vi "Settings Dialog.vi"(11 "settings in":T1={"sample rate"=100.0, "input range"=10.0, "logfile path"=path "", "Simulated Signal"={"signal type"=enum."Sine Wave", "frequency"=1000.0, "amplitude"=5.0}} {"Simulated Signal"."amplitude" format="%.0pV"; "Simulated Signal"."frequency" format="%.2pHz"; "input range" format="%.0pV"; "sample rate" format="%.2pHz"}) -> (1 "cancelled":bool, 3 "settings out":T1={"sample rate"=100.0, "input range"=10.0, "logfile path"=path "", "Simulated Signal"={"signal type"=enum."Sine Wave", "frequency"=1000.0, "amplitude"=5.0}} {"Simulated Signal"."amplitude" format="%.0pV"; "Simulated Signal"."frequency" format="%.2pHz"; "input range" format="%.0pV"; "sample rate" format="%.2pHz"})   [LabVIEW 2023]
doc: "Dialog for obtaining data acquisition & logging settings."
uses:
  Measure and Log Settings.ctl
  Simulated Signal Type.ctl
panel:
  in  "Simulated Signal":T3={"type"=0, "frequency"=1000.0, "amplitude"=5.0} {"amplitude" format="%.0pV"; "frequency" format="%.2pHz"; "type" items=["Sine Wave", "Square Wave with Noise"]}
  in  "Input Range":dbl=10.0 format="%.0pV"
  in  "Log File Base Path":path
  in  "Cancel Button":bool
  in  "OK Button":bool
  in  "Sample Period":dbl=0.01 format="%.2ps"
  in  "Sample Rate":dbl=100.0 format="%.2pHz"
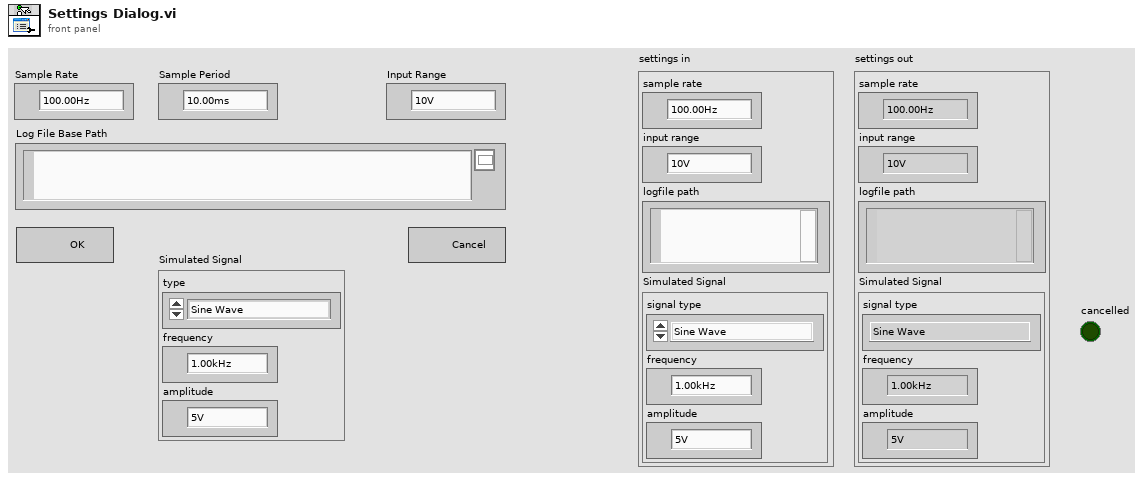
[diagram p1: front panel]
types:
  T1 = typedef "Measure and Log Settings.ctl" = cluster{"sample rate":dbl, "input range":dbl, "logfile path":path, "Simulated Signal":cluster{"signal type":T2, "frequency":dbl, "amplitude":dbl}}
  T2 = typedef "Simulated Signal Type.ctl" = enum16{"Sine Wave", "Square Wave with Noise"}
  T3 = cluster{"type":u16, "frequency":dbl, "amplitude":dbl}
  T4 = cluster{"signal type":T2, "frequency":dbl, "amplitude":dbl}
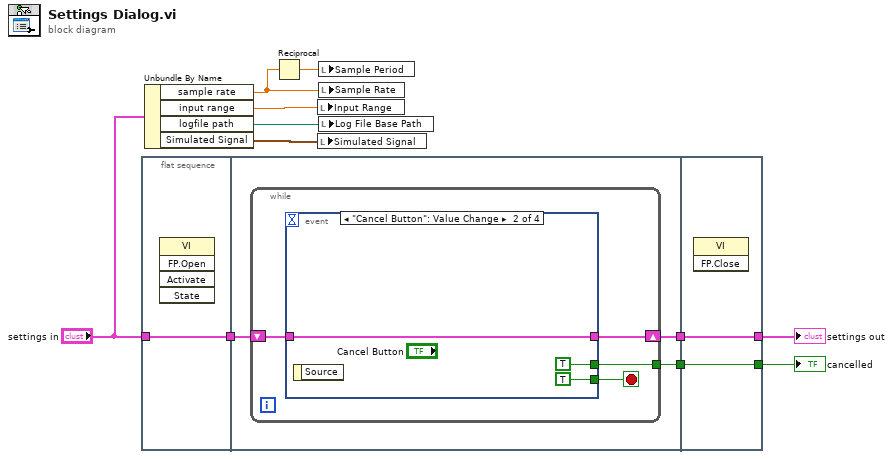
[diagram p0: block diagram]
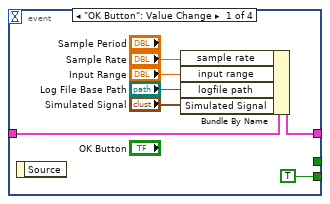
[diagram p2: hidden frame]
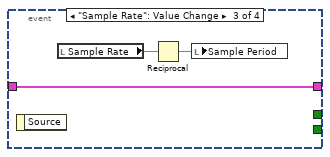
[diagram p3: hidden frame]
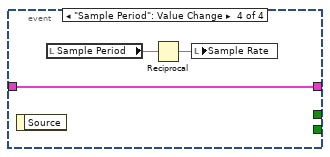
[diagram p4: hidden frame]
diagram:
  n1 = flat-sequence {
    tunnel: [w12] -> w7
    tunnel: "settings in" -> [w12]
    tunnel: [w15] -> w10
    tunnel: [w14] -> w8
    tunnel: w7 -> [w13]
    tunnel: [w37] -> w11
    tunnel: w10 -> [w37]
    tunnel: [w36] -> w9
    tunnel: w8 -> [w36]
    frame #0 {
      n2 = invoke class="VI" method="FP.Open"() -> ()  [unwired: 5 in, 5 out]
    }
    frame #1 {
      n3 = while {
        tunnel: [w19] -> w15
        shift-right: [w18] -> w14
        shift-left: w13 -> [w17]
        stop <- w16 stop-if-true
        n4 = event shown="[1] \"Cancel Button\": Value Change" {
          selector: _ -> [_ _ _ _]
          dyn-events: _ -> [_ _ _ _]
          timeout: _ -> [_ _ _ _]
          tunnel: [_ TRUE _ _] -> w19
          tunnel: [w25 w28 w30 w35] -> w18
          tunnel: w17 -> [w26 w28 w30 w35]
          tunnel: [TRUE TRUE _ _] -> w16
          event "OK Button": Value Change {
            n5 = event-data() -> ()  [unwired: 1 in, 1 out]
            n6 = Bundle By Name(cluster=w26, "sample rate"="Sample Rate", "input range"="Input Range", "logfile path"="Log File Base Path", "Simulated Signal"="Simulated Signal") -> (w25:T1)
          }
          event "Cancel Button": Value Change {
            n7 = event-data() -> ()  [unwired: 1 in, 1 out]
          }
          event "Sample Rate": Value Change {
            n8 = event-data() -> ()  [unwired: 1 in, 1 out]
            n9 = local read "Sample Rate"() -> (w32:dbl)
            n10 = Reciprocal(x=w32) -> (1/x=w31:dbl)
            n11 = local write "Sample Period"(w31) -> ()
          }
          event "Sample Period": Value Change {
            n12 = event-data() -> ()  [unwired: 1 in, 1 out]
            n13 = local read "Sample Period"() -> (w34:dbl)
            n14 = Reciprocal(x=w34) -> (1/x=w33:dbl)
            n15 = local write "Sample Rate"(w33) -> ()
          }
        }
      }
    }
    frame #2 {
      n16 = invoke class="VI" method="FP.Close"() -> ()  [unwired: 3 in, 3 out]
    }
  }
  n17 = Unbundle By Name("settings in") -> ("sample rate"=w2:dbl, "input range"=w5:dbl, "logfile path"=w4:path, "Simulated Signal"=w3:T4)
  n18 = Reciprocal(x=w2) -> (1/x=w1:dbl)
  n19 = local write "Input Range"(w5) -> ()
  n20 = local write "Simulated Signal"(w3) -> ()
  n21 = local write "Sample Period"(w1) -> ()
  n22 = local write "Sample Rate"(w2) -> ()
  n23 = local write "Log File Base Path"(w4) -> ()
  "settings out" <- w9
  "cancelled" <- w11
